vi "set_duty.vi"(8 "error in (no error)":errorcluster, 10 "Duty":dbl, 11 "VISA Refnum in":refnum<visa-resource-name>) -> (0 "error out":errorcluster, 3 "VISA Refnum out":refnum<visa-resource-name>)   [LabVIEW 2021]
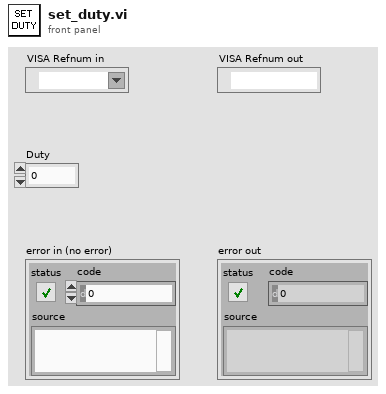
[diagram p1: front panel]
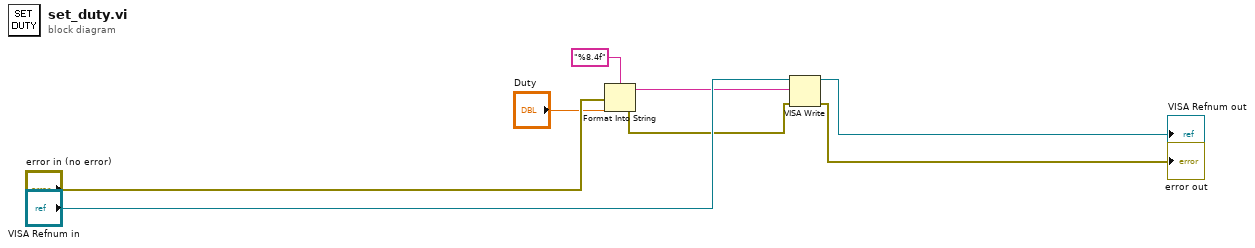
[diagram p0: block diagram]
diagram:
  n1 = Format Into String(format string="%8.4f", error in="error in (no error)", "Duty") -> (resulting string=w4:string, error out=w3:errorcluster)  [unwired: 1 in]
  n2 = VISA Write(VISA resource name="VISA Refnum in", write buffer=w4, error in (no error)=w3) -> (VISA resource name out=→"VISA Refnum out":refnum<visa-resource-name>, error out=→"error out":errorcluster)  [unwired: 1 out]
